vi "RT Loop - Data Acquisition and Logging.vi"(8 "error in (no error)":errorcluster caption="错误输入（无错误）", 9 "Acquisition and Logging Configuration":T1={"Samples per Read"=100, "Number of Reads to Save"=20, "Number of Channels"=4, "Channel Scale Array"=[1.0, 1.0, 1.0, 1.0], "Channel Names"=["Mod\\AI0", "Mod\\AI1", "Mod\\AI2", "Mod\\AI3"], "Trigger - RMS Value"=0.9999999999999994, "Trigger - Channel"=0, "Trigger - Time (Minute)"=10, "TDMS Properties"=[{"Name"="Company", "Value"="TongRui"}, {"Name"="Developer", "Value"="SUN"}], "Data File Name"="cRIO_Data", "Date Rate"=20} caption="采集与记录配置" {"Date Rate" items=["51.200 kS/s (NI 9234)"=1, "25.600 kS/s (NI 9234)"=2, "17.067 kS/s (NI 9234)"=3, "12.80 kS/s (NI 9234)"=4, "10.240 kS/s (NI 9234)"=5, "8.533 kS/s (NI 9234)"=6, "7.314 kS/s (NI 9234)"=7, "6.400 kS/s (NI 9234)"=8, "5.689 kS/s (NI 9234)"=9, "5.120 kS/s (NI 9234)"=10, "4.654 kS/s (NI 9234)"=11, "4.267 kS/s (NI 9234)"=12, "3.938 kS/s (NI 9234)"=13, "3.657 kS/s (NI 9234)"=14, "3.413 kS/s (NI 9234)"=15, "3.200 kS/s (NI 9234)"=16, "3.012 kS/s (NI 9234)"=17, "2.845 kS/s (NI 9234)"=18, "2.695 kS/s (NI 9234)"=19, "2.560 kS/s (NI 9234)"=20, "2.438 kS/s (NI 9234)"=21, "2.328 kS/s (NI 9234)"=22, "2.226 kS/s (NI 9234)"=23, "2.133 kS/s (NI 9234)"=24, "2.048 kS/s (NI 9234)"=25, "1.969 kS/s (NI 9234)"=26, "1.896 kS/s (NI 9234)"=27, "1.829 kS/s (NI 9234)"=28, "1.765 kS/s (NI 9234)"=29, "1.707 kS/s (NI 9234)"=30, "1.652 kS/s (NI 9234)"=31]}, 10 "Acquisition and Logging Queue":refnum<queue> caption="采集与记录队列", 11 "Message Queue":refnum<queue> caption="消息队列") -> (3 "State History":string caption="状态历史")   [LabVIEW 2013]
uses:
  support/Message Queue/Message Cluster.ctl
  controls/Acquisition and Logging Configuration.ctl
  controls/TDMS Properties.ctl
  <vilib>/LabVIEW Targets/FPGA/cRIO/shared/nicrio_ModuleControls/nicrio_cRIO-9234_DataRatesRing2.ctl
  controls/FPGA VI Reference.ctl
  Globals/Global - Configuration Options.vi
  Globals/Global - Monitoring Variables.vi
  support/Message Queue/Message Queue.lvlib
panel:
  # "通道"
  # "保存"
  # "采样"
  # "触发"
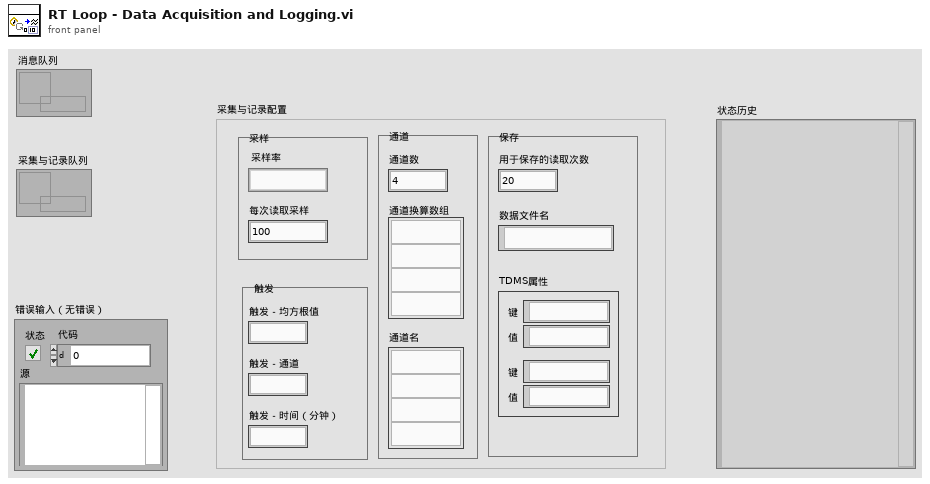
[diagram p1: front panel]
types:
  T1 = typedef "Acquisition and Logging Configuration.ctl" = cluster{"Samples per Read":i32, "Number of Reads to Save":i32, "Number of Channels":i32, "Channel Scale Array":fxp<+,24,12>[], "Channel Names":string[], "Trigger - RMS Value":dbl, "Trigger - Channel":i32, "Trigger - Time (Minute)":i32, "TDMS Properties":T2[], "Data File Name":string, "Date Rate":T3}
  T2 = typedef "TDMS Properties.ctl" = cluster{"Name":string, "Value":string}
  T3 = typedef "nicrio_cRIO-9234_DataRatesRing2.ctl" = u16
  T4 = typedef "FPGA VI Reference.ctl" = refnum<k20>
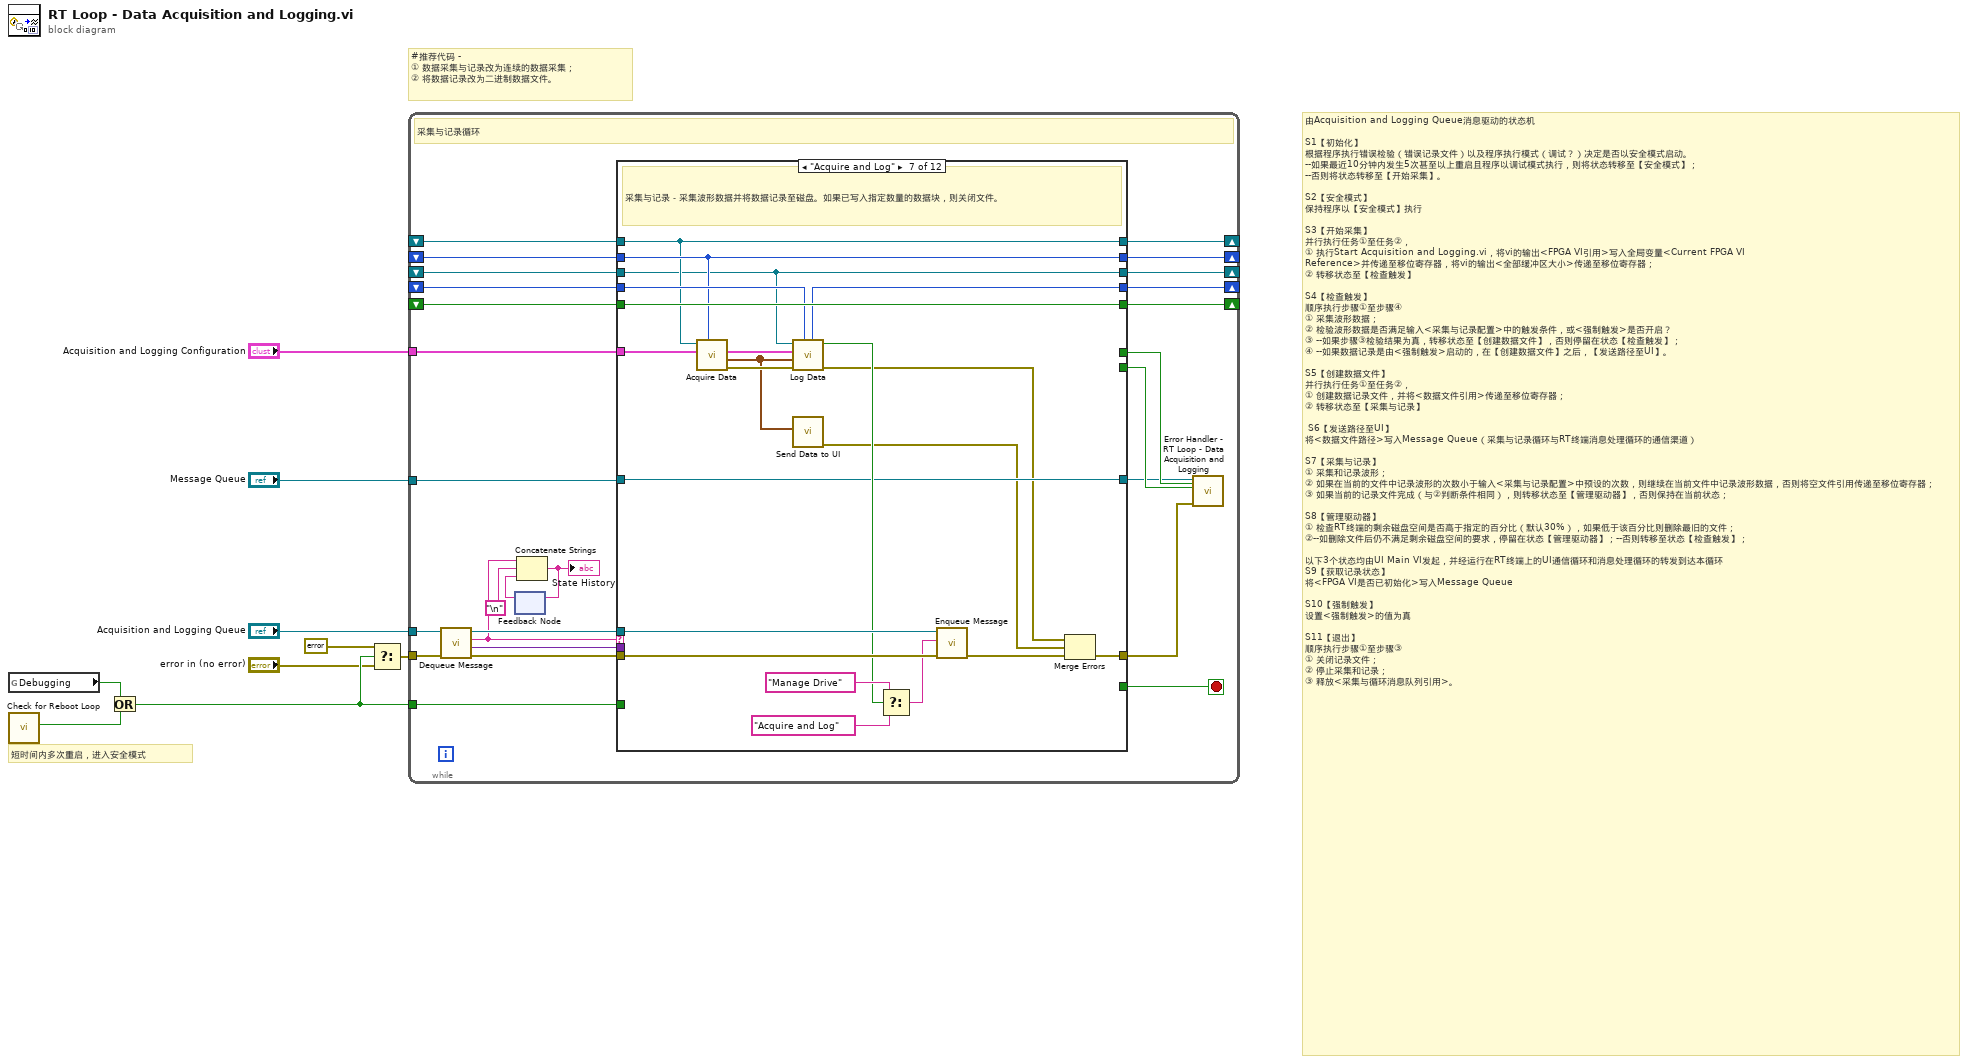
[diagram p0: block diagram]
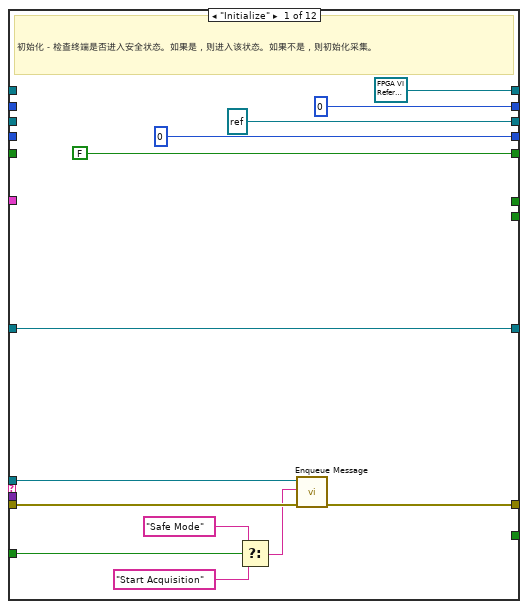
[diagram p2: hidden frame]
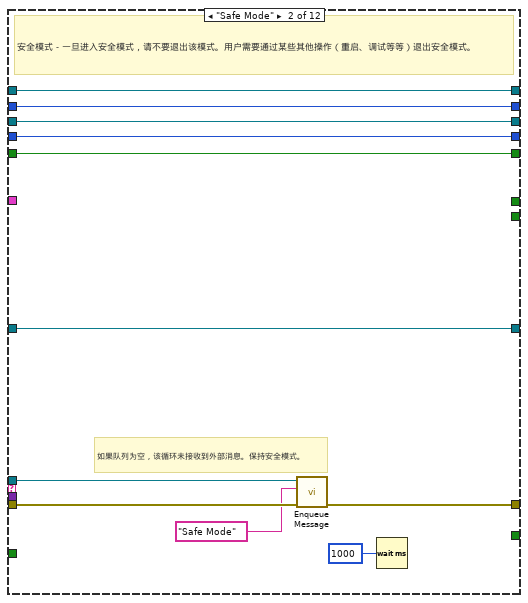
[diagram p3: hidden frame]
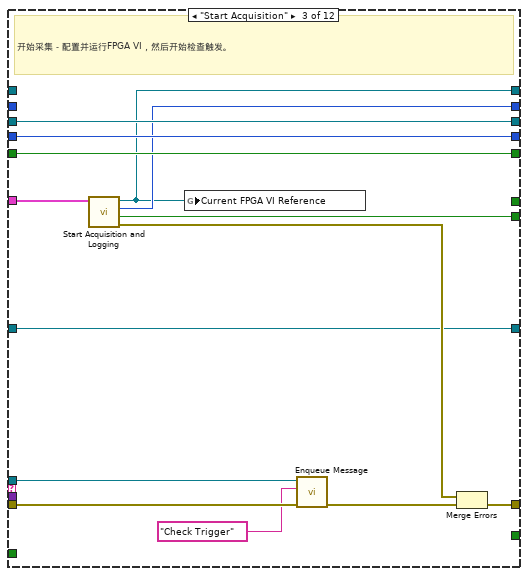
[diagram p4: hidden frame]
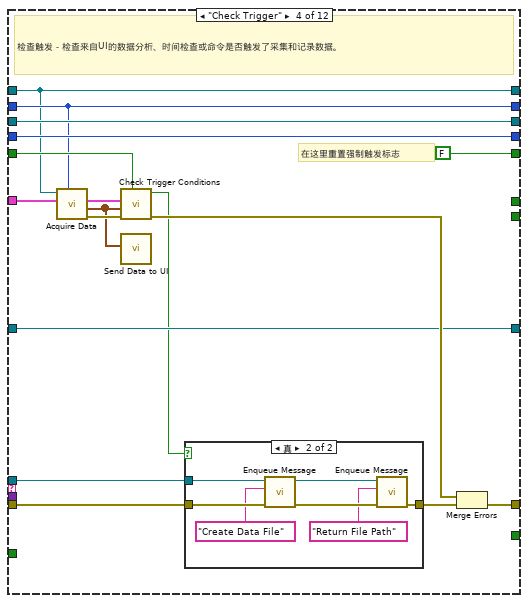
[diagram p5: hidden frame]
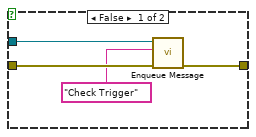
[diagram p6: hidden frame]
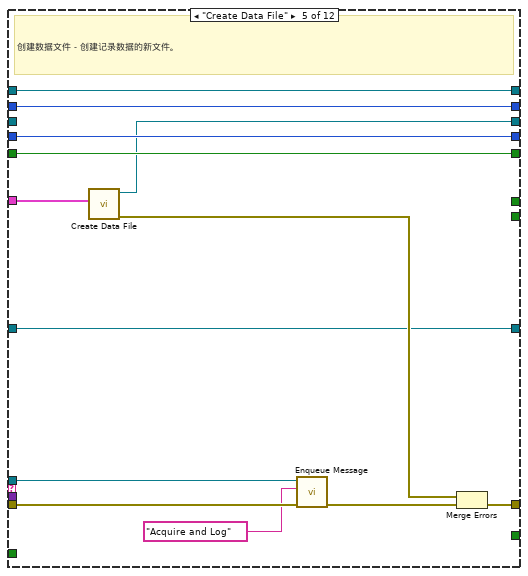
[diagram p7: hidden frame]
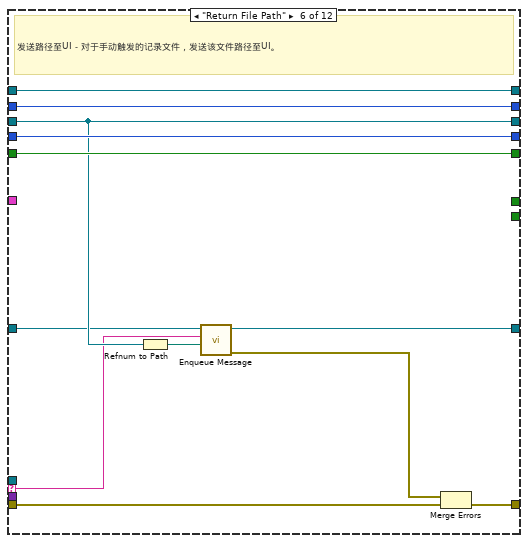
[diagram p8: hidden frame]
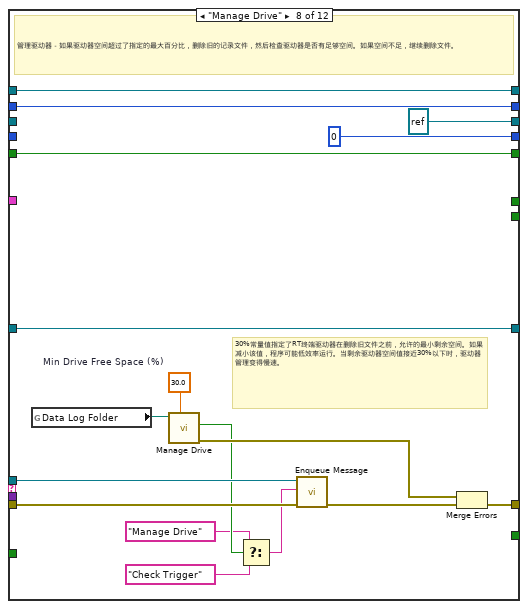
[diagram p9: hidden frame]
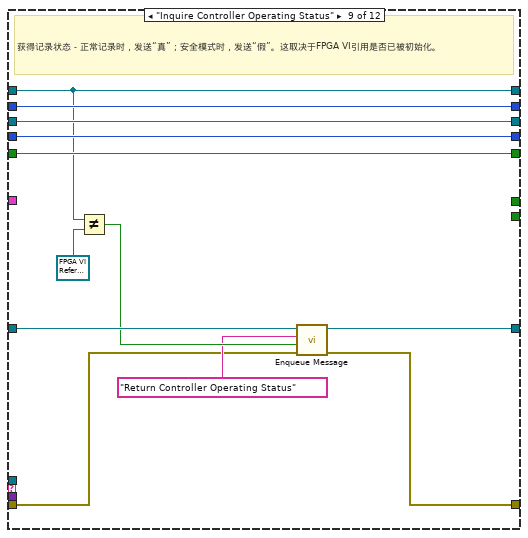
[diagram p10: hidden frame]
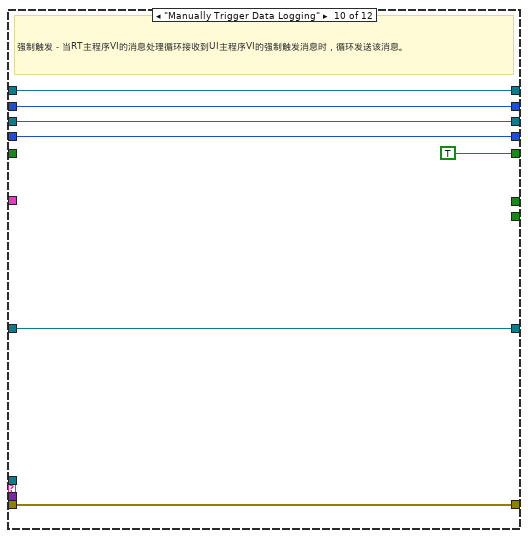
[diagram p11: hidden frame]
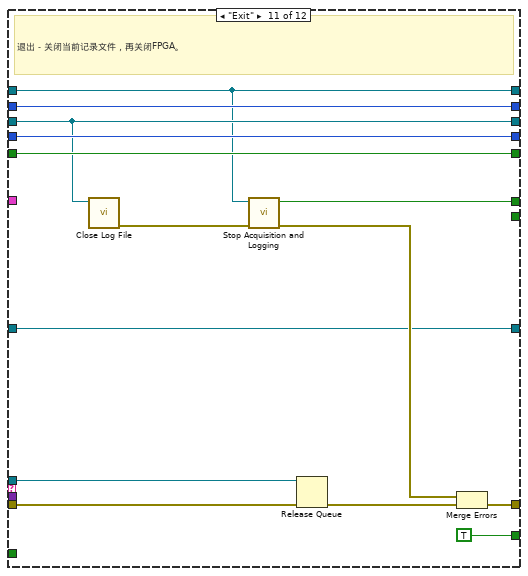
[diagram p12: hidden frame]
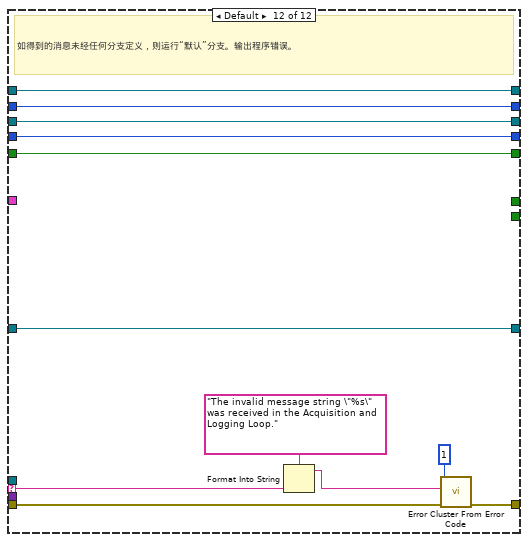
[diagram p13: hidden frame]
diagram:
  # "#推荐代码 - \n① 数据采集与记录改为连续的数据采集；\n② 将数据记录改为二进制数据文件。"
  # "由Acquisition and Logging Queue消息驱动的状态机\n\nS1【初始化】\n根据程序执行错误检验（错误记录文件）以及程序执行模式（调试？）决定是否以安全模式启动。\n--如果最近10分钟内发生5次甚至以上重启且程序以调试模式执行，则将状态转移至【安全模式】；\n--否则将状态转移至【开始采集】。\n\nS2【安全模式】\n保持程序以【安全模式】执行\n\nS3【开始采集】\n并行执行任务①至任务②，\n① 执行Start Acquisition and Logging.vi，将vi的输出<FPGA VI引用>写入全局变量<Current FPGA VI Reference>并传递至移位寄存器，将vi的输出<全部缓冲区大小>传递至移位寄存器；\n② 转移状态至【检查触发】\n\nS4【检查触发】\n顺序执行步骤①至步骤④\n① 采集波形数据；\n② 检验波形数据是否满足输入<采集与记录配置>中的触发条件，或<强制触发>是否开启？\n③ --如果步骤③检验结果为真，转移状态至【创建数据文件】，否则停留在状态【检查触发】；\n④ --如果数据记录是由<强制触发>启动的，在【创建数据文件】之后，【发送路径至UI】。\n\nS5【创建数据文件】\n并行执行任务①至任务②，\n① 创建数据记录文件，并将<数据文件引用>传递至移位寄存器；\n② 转移状态至【采集与记录】\n\n S6【发送路径至UI】\n将<数据文件路径>写入Message Queue（采集与记录循环与RT终端消息处理循环的通信渠道）\n\nS7【采集与记录】\n① 采集和记录波形；\n② 如果在当前的文件中记录波形的次数小于输入<采集与记录配置>中预设的次数，则继续在当前文件中记录波形数据，否则将空文件引用传递至移位寄存器；\n③ 如果当前的记录文件完成（与②判断条件相同），则转移状态至【管理驱动器】，否则保持在当前状态；\n\nS8【管理驱动器】\n① 检查RT终端的剩余磁盘空间是否高于指定的百分比（默认30%），如果低于该百分比则删除最旧的文件；\n②--如删除文件后仍不满足剩余磁盘空间的要求，停留在状态【管理驱动器】；--否则转移至状态【检查触发】；\n\n以下3个状态均由UI Main VI发起，并经运行在RT终端上的UI通信循环和消息处理循环的转发到达本循环\nS9【获取记录状态】\n将<FPGA VI是否已初始化>写入Message Queue\n\nS10【强制触发】\n设置<强制触发>的值为真\n\nS11【退出】\n顺序执行步骤①至步骤③\n① 关闭记录文件；\n② 停止采集和记录；\n③ 释放<采集与循环消息队列引用>。"
  # "短时间内多次重启，进入安全模式"
  n1 = global read "Global - Configuration Options.vi" "Debugging"() -> (w4:bool)
  n2 = call "Check for Reboot Loop.vi"() -> ("Start in Safe Mode?"=w5:bool)  [unwired: 10 in, 1 out]
  n3 = Or(x=w4, y=w5) -> (x .or. y?=w3:bool)
  n4 = Select(t=errorcluster {"status"=FALSE, "code"=0, "source"=""}, s=w3, f="error in (no error)") -> (s? t:f=w6:errorcluster)
  n5 = while {
    tunnel: "Acquisition and Logging Queue" -> [w33]
    tunnel: "Message Queue" -> [w18]
    shift-right: [w28] -> _
    shift-left: _ -> [w30]
    shift-right: [w27] -> _
    shift-left: _ -> [w29]
    tunnel: "Acquisition and Logging Configuration" -> [w26]
    shift-right: [w23] -> _
    shift-left: _ -> [w24]
    shift-right: [w21] -> _
    shift-left: _ -> [w22]
    shift-right: [w19] -> _
    shift-left: _ -> [w20]
    tunnel: w6 -> [w16]
    tunnel: w3 -> [w15]
    stop <- w36 stop-if-true
    # "采集与记录循环"
    n6 = call "Dequeue Message.vi"("error in (no error)"=w16, "Message Queue"=w33) -> ("error out"=w35:errorcluster, "Message Data"=w34:variant, "Message"=w11:string, "dup Message Queue"=w31:refnum<queue>)  [unwired: 6 in]
    n7 = feedback #1() -> (w10:string)  [unwired: 1 in]
    n8 = Concatenate Strings(w11, "\n", w10) -> (w13:string)
    "State History" <- w13
    n9 = feedback-in #1(w13) -> ()
    n10 = case "Message Cases" shown="\"Acquire and Log\"" w11 {
      selector: w11 -> [_ _ _ _ _ w120 _ _ _ _ _ w209]
      tunnel: w31 -> [w48 w57 w68 w85 w110 _ w145 w159 _ _ w198 _]
      tunnel: w35 -> [w49 w58 w74 w91 w114 w127 w148 w165 w166 w184 w194 w200]
      tunnel: [w44 w56 w72 w90 w113 w118 w147 w162 w170 w184 w195 w207] -> w32
      tunnel: [_ _ _ _ _ _ _ _ _ _ TRUE _] -> w36
      tunnel: w34 -> [_ _ _ _ _ _ _ _ _ _ _ _]
      tunnel: w30 -> [_ w60 _ w77 w115 w126 w130 w164 w173 w183 w185 w205]
      tunnel: w29 -> [_ w59 _ w79 w112 w125 w134 w163 w177 w182 w193 w204]
      tunnel: [T4 refnum ("FPGA VI Reference") w60 w61 w77 w115 w126 w130 w164 w173 w183 w185 w205] -> w28
      tunnel: [0 ("Total Buffer Size") w59 w62 w79 w112 w125 w134 w163 w177 w182 w193 w204] -> w27
      tunnel: w26 -> [_ _ w73 w89 w107 _ w137 _ _ _ _ _]
      tunnel: [_ _ w70 _ _ _ _ _ _ _ _ _] -> w25
      tunnel: w24 -> [_ w55 w66 w80 w108 w124 w144 w152 w176 _ w191 w203]
      tunnel: [FALSE ("Force Trigger Flag") w55 w66 FALSE ("Force Trigger Flag") w108 w124 w144 w152 w176 TRUE ("Force Trigger Flag") w191 w203] -> w23
      tunnel: w22 -> [_ w54 w65 w84 _ w122 w129 _ w175 w181 w188 w202]
      tunnel: [refnum<k34> refnum ("Current Log File") w54 w65 w84 w103 w122 w129 refnum<k34> refnum ("t") w175 w181 w188 w202] -> w21
      tunnel: w20 -> [_ w53 w64 w83 w105 w123 w138 _ w174 w179 w190 w201]
      tunnel: [0 ("Number of Blocks Saved") w53 w64 w83 w105 w123 w128 0 ("Number of Blocks Saved") w174 w179 w190 w201] -> w19
      tunnel: w18 -> [w42 w51 w63 w78 w104 w119 w139 w150 w171 w178 w186 w199]
      tunnel: [_ _ _ _ _ _ _ _ _ _ w187 _] -> w17
      tunnel: w15 -> [w43 _ _ _ _ _ _ _ _ _ _ _]
      tunnel: [w42 w51 w63 w78 w104 w116 w139 w150 w167 w178 w186 w199] -> w14
      frame "Initialize" {
        # "初始化－检查终端是否进入安全状态。如果是，则进入该状态。如果不是，则初始化采集。"
        n11 = Select(t="Safe Mode", s=w43, f="Start Acquisition") -> (s? t:f=w45:string)
        n12 = call "Enqueue Message.vi"("error in (no error)"=w49, "Message"=w45, "Message Queue"=w48) -> ("error out"=w44:errorcluster)  [unwired: 7 in, 1 out]
      }
      frame "Safe Mode" {
        # "如果队列为空，该循环未接收到外部消息。保持安全模式。"
        # "安全模式－一旦进入安全模式，请不要退出该模式。用户需要通过某些其他操作（重启、调试等等）退出安全模式。"
        n13 = call "Enqueue Message.vi"("error in (no error)"=w58, "Message"="Safe Mode", "Message Queue"=w57) -> ("error out"=w56:errorcluster)  [unwired: 7 in, 1 out]
        n14 = Wait (ms)(milliseconds to wait=u32 1000 ("等待时间（毫秒）")) -> ()  [unwired: 1 out]
      }
      frame "Start Acquisition" {
        # "开始采集－配置并运行FPGA VI，然后开始检查触发。"
        n15 = call "Start Acquisition and Logging.vi"("Acquisition and Logging Configuration"=w73) -> ("error out"=w71:errorcluster, "Wait on IRQ Timeout?"=w70:bool, "Total Buffer Size"=w62:i32, "FPGA VI Reference"=w61:T4)  [unwired: 7 in]
        n16 = global write "Global - Monitoring Variables.vi" "Current FPGA VI Reference"(w61) -> ()
        n17 = call "Enqueue Message.vi"("error in (no error)"=w74, "Message"="Check Trigger", "Message Queue"=w68) -> ("error out"=w69:errorcluster)  [unwired: 7 in, 1 out]
        n18 = Merge Errors(w71, w69) -> (w72:errorcluster)
      }
      frame "Check Trigger" {
        # "在这里重置强制触发标志"
        # "检查触发－检查来自UI的数据分析、时间检查或命令是否触发了采集和记录数据。"
        n19 = call "Acquire Data.vi"("Total Buffer Size"=w79, "Acquisition and Logging Configuration"=w89, "FPGA VI Reference"=w77) -> ("error out"=w87:errorcluster, "Waveform Data"=w75:waveform(sgl)[], "dup Acquisition and Logging Configuration"=w86:T1)  [unwired: 6 in]
        n20 = call "Check Trigger Conditions.vi"("Force Trigger?"=w80, "error in (no error)"=w87, "Waveform Data"=w75, "Acquisition and Logging Configuration"=w86) -> ("error out"=w88:errorcluster, "Trigger Condition Met?"=w76:bool)  [unwired: 6 in]
        n21 = call "Send Data to UI.vi"("Waveform Data Array"=w75) -> ()  [unwired: 10 in, 1 out]
        n22 = case shown="真" w76 {
          tunnel: w91 -> [w95 w102]
          tunnel: [w94 w98] -> w81
          tunnel: w85 -> [w93 w101]
          frame False {
            n23 = call "Enqueue Message.vi"("error in (no error)"=w95, "Message"="Check Trigger", "Message Queue"=w93) -> ("error out"=w94:errorcluster)  [unwired: 7 in, 1 out]
          }
          frame True {
            n24 = call "Enqueue Message.vi"("error in (no error)"=w102, "Message"="Create Data File", "Message Queue"=w101) -> ("error out"=w99:errorcluster, "dup Message Queue"=w97:refnum<queue>)  [unwired: 7 in]
            n25 = call "Enqueue Message.vi"("error in (no error)"=w99, "Message"="Return File Path", "Message Queue"=w97) -> ("error out"=w98:errorcluster)  [unwired: 7 in, 1 out]
          }
        }
        n26 = Merge Errors(w88, w81) -> (w90:errorcluster)
      }
      frame "Create Data File" {
        # "创建数据文件－创建记录数据的新文件。"
        n27 = call "Create Data File.vi"("Acquisition and Logging Configuration"=w107) -> ("error out"=w106:errorcluster, "TDMS File Reference"=w103:refnum<k34>)  [unwired: 9 in]
        n28 = call "Enqueue Message.vi"("error in (no error)"=w114, "Message"="Acquire and Log", "Message Queue"=w110) -> ("error out"=w111:errorcluster)  [unwired: 7 in, 1 out]
        n29 = Merge Errors(w106, w111) -> (w113:errorcluster)
      }
      frame "Return File Path" {
        # "发送路径至UI－对于手动触发的记录文件，发送该文件路径至UI。"
        n30 = Refnum to Path(1:w122) -> (0:w121:path)
        n31 = call "Enqueue Message.vi"("Message Data"=w121, "Message"=w120, "Message Queue"=w119) -> ("error out"=w117:errorcluster, "dup Message Queue"=w116:refnum<queue>)  [unwired: 7 in]
        n32 = Merge Errors(w117, w127) -> (w118:errorcluster)
      }
      frame "Acquire and Log" {
        # "采集与记录－采集波形数据并将数据记录至磁盘。如果已写入指定数量的数据块，则关闭文件。"
        n33 = call "Acquire Data.vi"("Total Buffer Size"=w134, "Acquisition and Logging Configuration"=w137, "FPGA VI Reference"=w130) -> ("error out"=w135:errorcluster, "Waveform Data"=w133:waveform(sgl)[], "dup Acquisition and Logging Configuration"=w136:T1)  [unwired: 6 in]
        n34 = call "Log Data.vi"("Number of Blocks Saved in"=w138, "error in (no error)"=w135, "Waveform Data Array"=w133, "Acquisition and Logging Configuration"=w136, "TDMS File Reference"=w129) -> ("error out"=w132:errorcluster, "Logging Complete?"=w140:bool, "Number of Blocks Saved out"=w128:i32)  [unwired: 4 in]
        n35 = call "Send Data to UI.vi"("Waveform Data Array"=w133) -> ("error out"=w131:errorcluster)  [unwired: 10 in]
        n36 = Select(t="Manage Drive", s=w140, f="Acquire and Log") -> (s? t:f=w141:string)
        n37 = call "Enqueue Message.vi"("error in (no error)"=w148, "Message"=w141, "Message Queue"=w145) -> ("error out"=w146:errorcluster)  [unwired: 7 in, 1 out]
        n38 = Merge Errors(w132, w131, w146) -> (w147:errorcluster)
      }
      frame "Manage Drive" {
        w161 = 30.0  # Min Drive Free Space (%)
        # "30%常量值指定了RT终端驱动器在删除旧文件之前，允许的最小剩余空间。如果减小该值，程序可能低效率运行。当剩余驱动器空间值接近30%以下时，驱动器管理变得慢速。"
        # "管理驱动器－如果驱动器空间超过了指定的最大百分比，删除旧的记录文件，然后检查驱动器是否有足够空间。如果空间不足，继续删除文件。"
        n39 = global read "Global - Configuration Options.vi" "Data Log Folder"() -> (w151:path)
        n40 = call "Manage Drive.vi"("Min Drive Free Space (%)"=w161, "Data Folder"=w151) -> ("error out"=w158:errorcluster, "Drive Space Below Limit"=w157:bool)  [unwired: 8 in]
        n41 = Select(t="Manage Drive", s=w157, f="Check Trigger") -> (s? t:f=w154:string)
        n42 = call "Enqueue Message.vi"("error in (no error)"=w165, "Message"=w154, "Message Queue"=w159) -> ("error out"=w160:errorcluster)  [unwired: 7 in, 1 out]
        n43 = Merge Errors(w158, w160) -> (w162:errorcluster)
      }
      frame "Inquire Controller Operating Status" {
        # "获得记录状态－正常记录时，发送“真”；安全模式时，发送“假”。这取决于FPGA VI引用是否已被初始化。"
        n44 = Not Equal?(x=w173, y=T4 refnum ("FPGA VI Reference")) -> (x != y?=w169:bool)
        n45 = call "Enqueue Message.vi"("error in (no error)"=w166, "Message Data"=w169, "Message"="Return Controller Operating Status", "Message Queue"=w171) -> ("error out"=w170:errorcluster, "dup Message Queue"=w167:refnum<queue>)  [unwired: 6 in]
      }
      frame "Manually Trigger Data Logging" {
        # "强制触发－当RT主程序VI的消息处理循环接收到UI主程序VI的强制触发消息时，循环发送该消息。"
      }
      frame "Exit" {
        # "退出－关闭当前记录文件，再关闭FPGA。"
        n46 = call "Close Log File.vi"("Log File"=w188) -> ("error out"=w189:errorcluster)  [unwired: 10 in]
        n47 = call "Stop Acquisition and Logging.vi"("error in (no error)"=w189, "FPGA VI Reference"=w185) -> ("error out"=w192:errorcluster, "Stop FPGA Timeout?"=w187:bool)  [unwired: 8 in]
        n48 = Release Queue(queue=w198, error in (no error)=w194) -> (error out=w196:errorcluster)  [unwired: 1 in, 2 out]
        n49 = Merge Errors(w192, w196) -> (w195:errorcluster)
      }
      frame Default {
        # "如得到的消息未经任何分支定义，则运行“默认”分支。输出程序错误。"
        n50 = Format Into String(format string="The invalid message string \"%s\" was received in the Acquisition and Logging Loop." ("Unknown Message Error Text"), w209) -> (resulting string=w206:string)  [unwired: 2 in, 1 out]
        n51 = call <vilib>:"Error Cluster From Error Code.vi"("error in (no error)"=w200, "error message (\"\")"=w206, "error code (0)"=1) -> ("error out"=w207:errorcluster)  [unwired: 6 in]
      }
    }
    n52 = call "Error Handler - RT Loop - Data Acquisition and Logging.vi"("Stop FPGA Timeout"=w17, "error in (no error)"=w32, "IRQ Timeout"=w25, "Message Queue"=w14) -> ()  [unwired: 7 in, 1 out]
  }
